vi "FilePackageReceive.vi"(8 "error in":errorcluster caption="错误输入（无错误）", 9 "PCFileLocation":string="C:\\Users\\Administrator\\Desktop\\Xmodem_2_FileReceive", 10 "PdFileLocation":string="/media/card/15CAG2018070200000025.key", 11 "ComIn":refnum<visa-resource-name>="COM16") -> (0 "error out":errorcluster caption="错误输出", 1 "Times":dbl, 2 "MD5":string, 3 "Result":bool, 4 "FileText":string, 5 "FileLen":u32)   [LabVIEW 2013]
uses:
  <vilib>/Instr/_visa.llb/VISA Flush IO Buffer Mask.ctl
  <vilib>/Instr/_visa.llb/VISA Set IO Buffer Mask.ctl
  RegisterPara.ctl
  <vilib>/Instr/_visa.llb/VISA Configure Serial Port (Instr).vi
  FileGolbalPara.vi
panel:
  out "数组":string[](array[string])
  out "MD5_2":string
  out "连接的字符串 2":string
  out "CRC？":bool
  out "文件内容":string
  out "读取缓冲区2":string
  out "连接的字符串":string
  out "FileName":string
  out "读取缓冲区":string
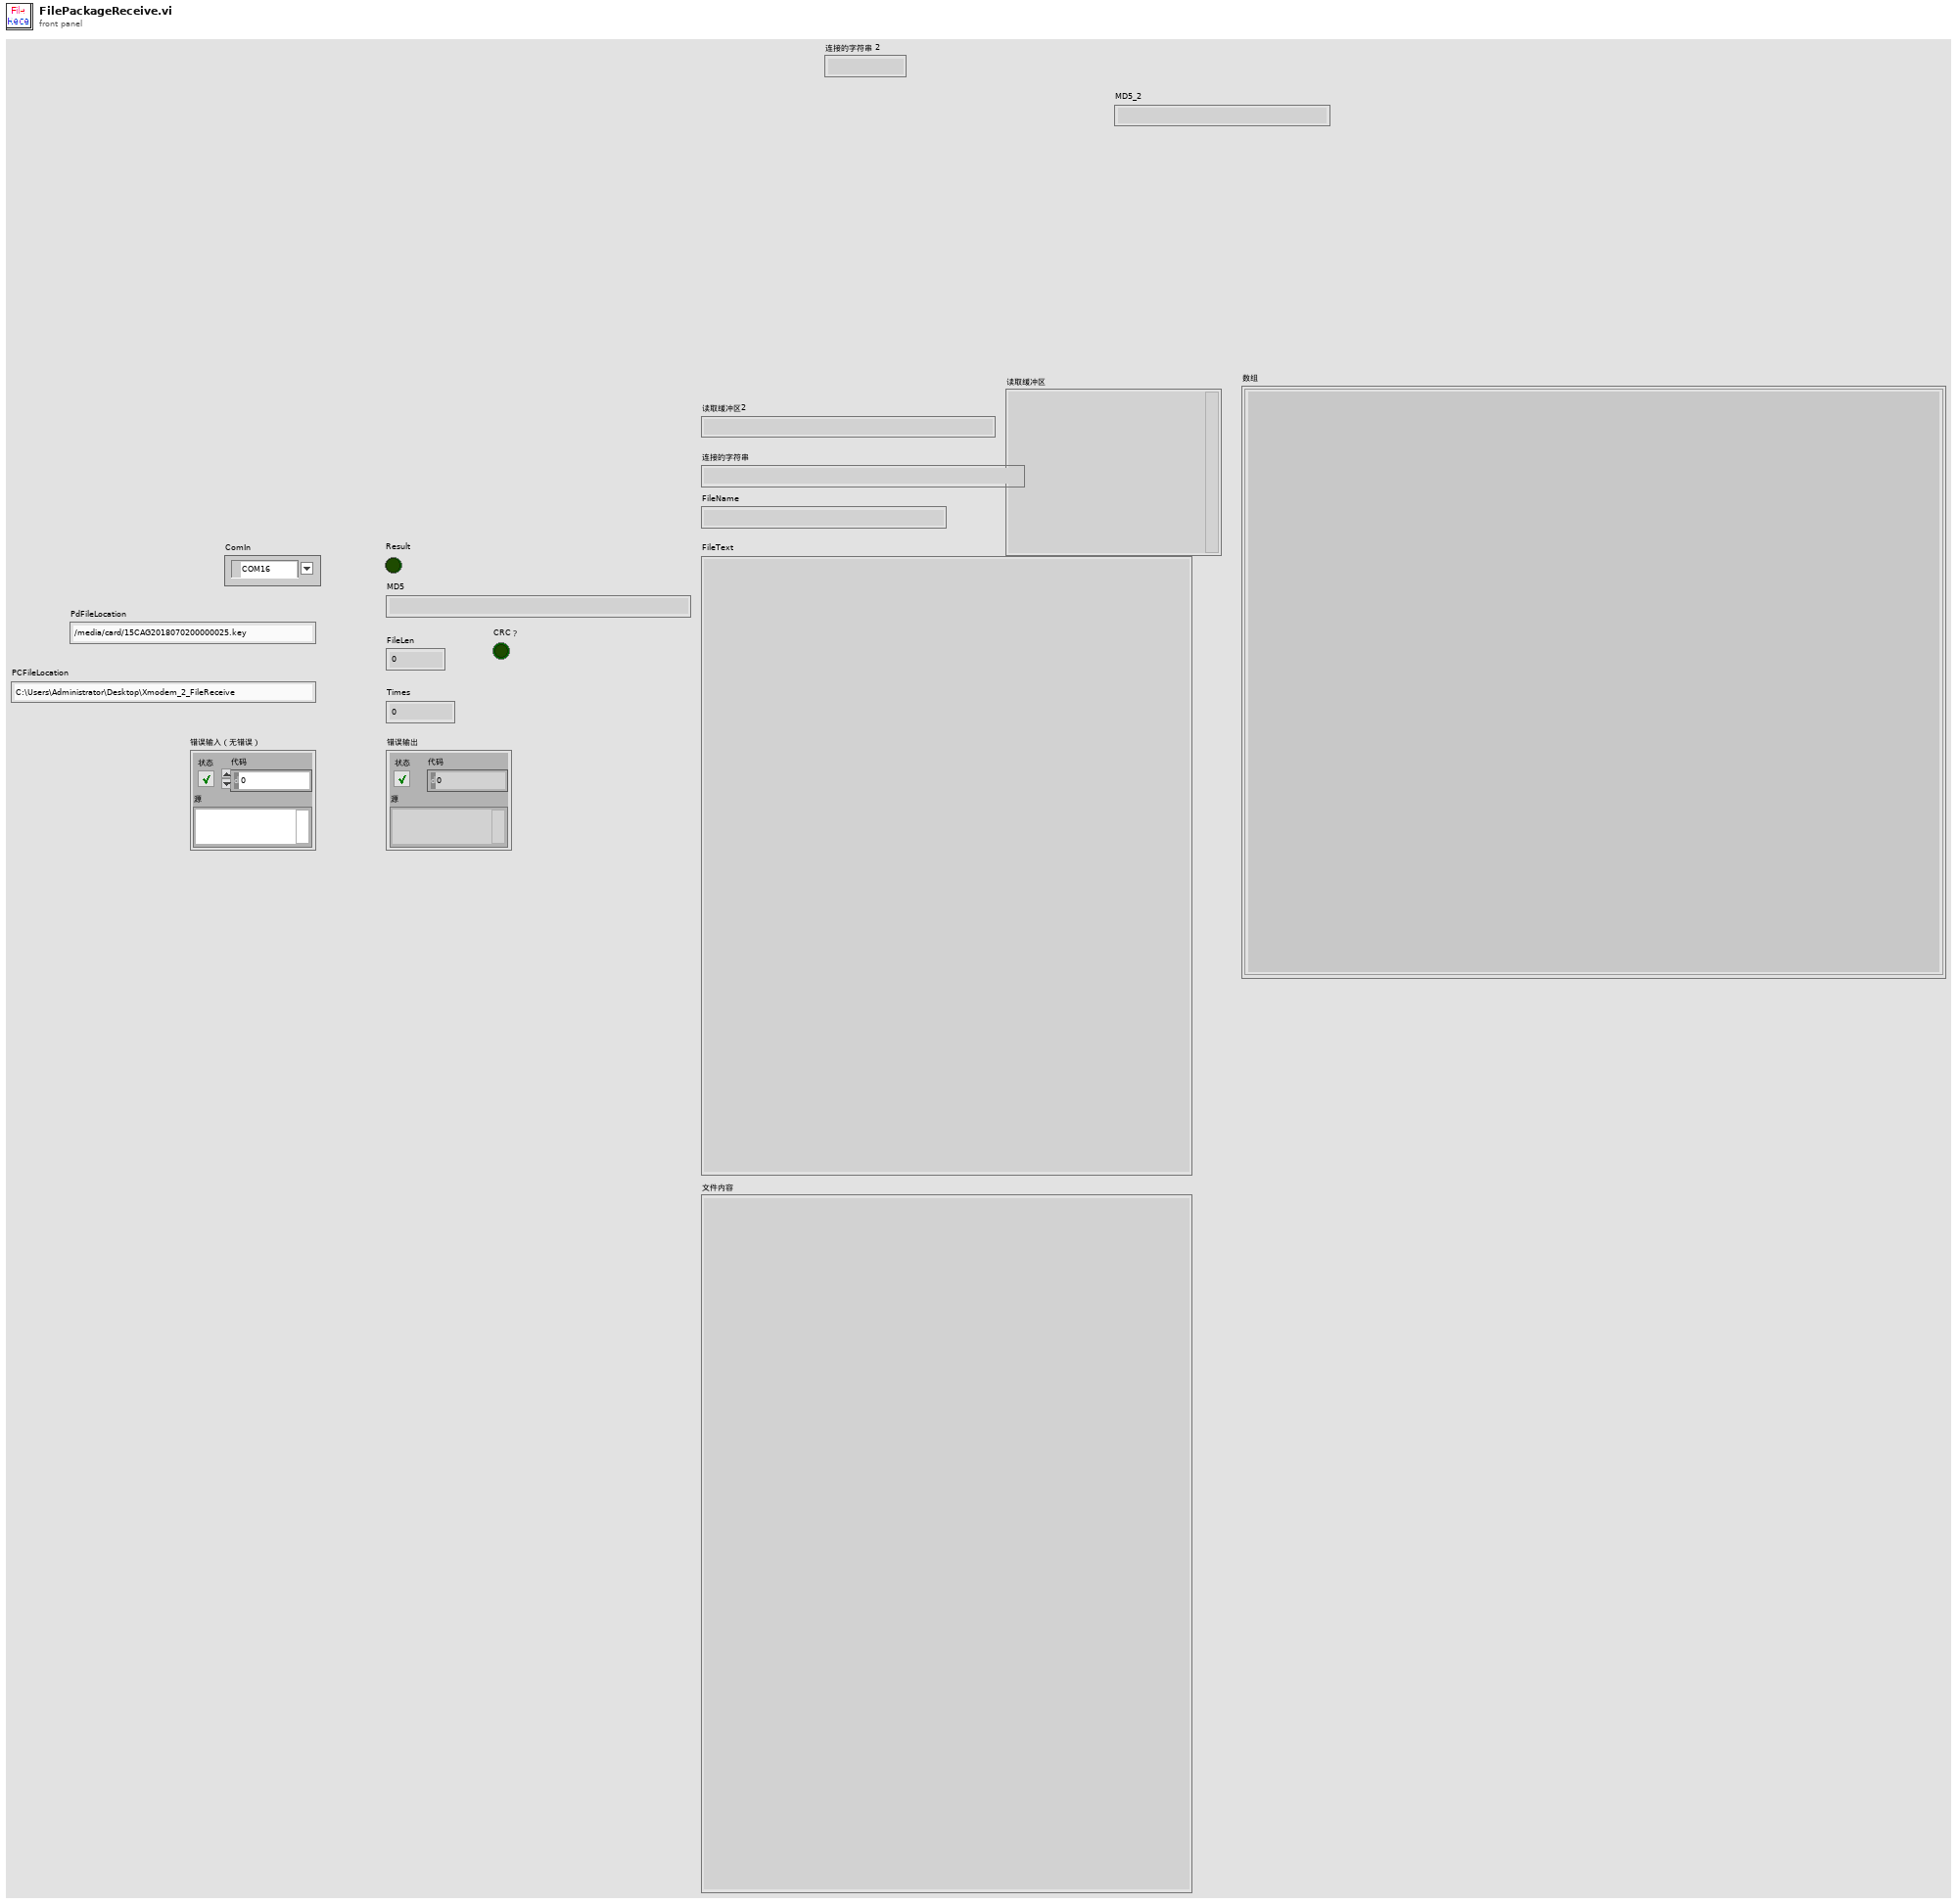
[diagram p1: front panel]
types:
  T1 = typedef "VISA Flush IO Buffer Mask.ctl" = u16
  T2 = cluster{"波特率":u32, "数据比特":u16, "奇偶":enum16{"None", "Odd", "Even", "Mark", "Space"}, "停止位":u16, "流控制":u16}
  T3 = typedef "RegisterPara.ctl" = cluster{"MD5":string, "文件总字节数":u32, "文件帧数":u32, "帧方式":enum16{"128K", "1024K-128K"}, "文件内容":string, "帧序号溢出标志":u32, "128包数":u32, "1024包数":u32}
  T4 = typedef "VISA Set IO Buffer Mask.ctl" = u16
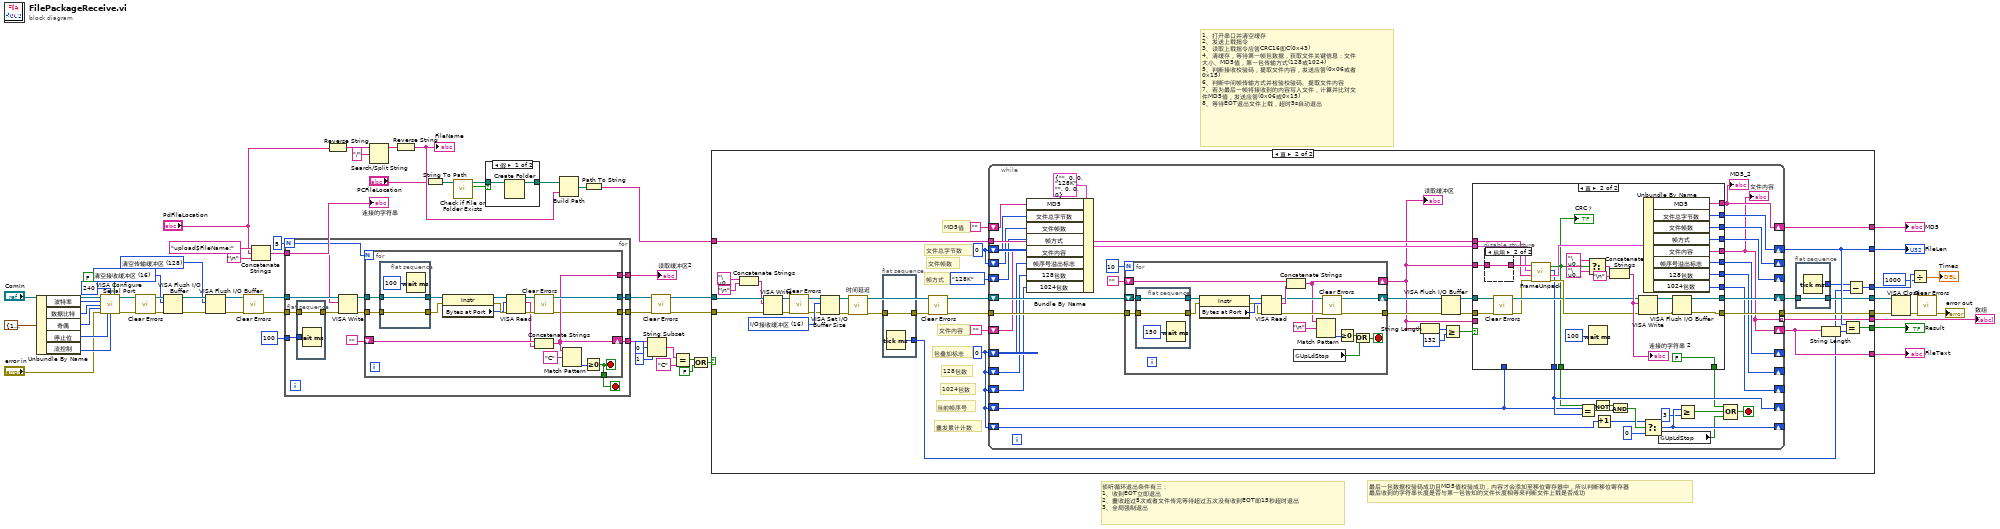
[diagram p0: block diagram]
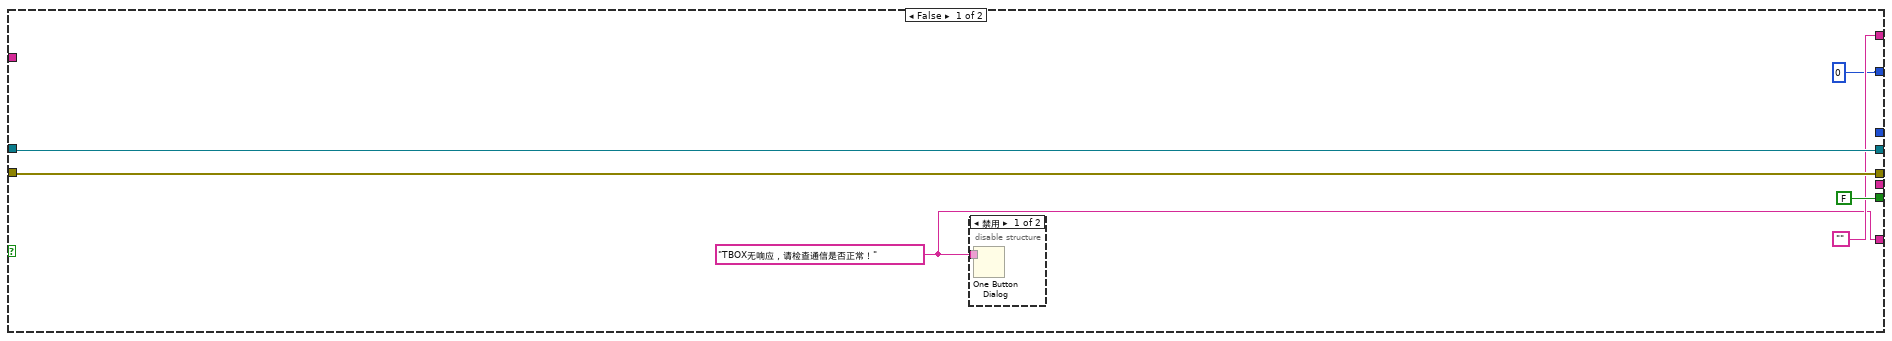
[diagram p3: hidden frame]
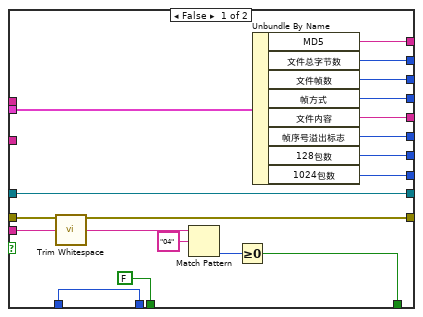
[diagram p5: hidden frame]
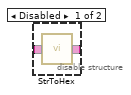
[diagram p6: hidden frame]
diagram:
  w48 = T1 128 items=["清空接收缓冲区"=16, "向设备写入传输缓冲区"=32, "清空接收缓冲区（无I/O）"=64, "清空传输缓冲区"=128] ("Mask")
  w52 = T1 16 items=["清空接收缓冲区"=16, "向设备写入传输缓冲区"=32, "清空接收缓冲区（无I/O）"=64, "清空传输缓冲区"=128] ("Mask")
  # "最后一包数据校验码成功且MD5值校验成功，内容才会添加至移位寄存器中，所以判断移位寄存器\n最后收到的字符串长度是否与第一包告知的文件长度相等来判断文件上载是否成功"
  # "侦听循环退出条件有三：\n1、收到EOT立即退出\n2、重收超过5次或者文件传完等待超过五次没有收到EOT即15秒超时退出\n3、全局强制退出"
  # "1、打开串口并清空缓存\n2、发送上载指令\n3、读取上载指令应答CRC16即C(0x43)\n4、清缓存，等待第一帧包数据，获取文件关键信息：文件\n大小、MD5值，第一包传输方式(128或1024)\n5、判断接收校验码，提取文件内容，发送应答(0x06或者\n0x15)\n6、判断中间帧传输方式并检验校验码、提取文件内容\n7、若为最后一帧将接收到的内容写入文件，计算并比对文\n件MD5值，发送应答(0x06或0x15)\n8、等待EOT退出文件上载，超时5s自动退出"
  n1 = Unbundle By Name(T2 {"波特率"=115200, "数据比特"=8, "奇偶"=enum."None", "停止位"=10, "流控制"=0} ("串口设置")) -> ("波特率"=w59:u32, "数据比特"=w58:u16, "奇偶"=w57:enum16{"None", "Odd", "Even", "Mark", "Space"}, "停止位"=w56:u16, "流控制"=w55:u16)
  n2 = call-poly "VISA Configure Serial Port"("VISA resource name"="ComIn", "termination char\n(0xA = '\\n' = LF)"=u8 240 ("termination char\n(0xA = '\\n' = LF)"), "Enable Termination\nChar (T)"=FALSE ("Enable Termination\nChar (T)"), "baud rate (9600)"=w59, "data bits (8)"=w58, "parity (0:none)"=w57, "error in (no error)"="error in", "stop bits (10: 1 bit)"=w56, "flow control (0:none)"=w55) -> ("VISA resource name out"=w53:refnum<visa-resource-name>, "error out"=w51:errorcluster)  [unwired: 5 in]
  n3 = call <vilib>:"Clear Errors.vi"("error in (no error)"=w51) -> ("error out"=w4:errorcluster)  [unwired: 6 in]
  n4 = VISA Flush I/O Buffer(VISA resource name=w53, mask (16)=w52, error in (no error)=w4) -> (VISA resource name out=w50:refnum<visa-resource-name>, error out=w49:errorcluster)
  n5 = VISA Flush I/O Buffer(VISA resource name=w50, mask (16)=w48, error in (no error)=w49) -> (VISA resource name out=w47:refnum<visa-resource-name>, error out=w46:errorcluster)
  n6 = call <vilib>:"Clear Errors.vi"("error in (no error)"=w46) -> ("error out"=w3:errorcluster)  [unwired: 6 in]
  n7 = Concatenate Strings("upload$FileName:", "PdFileLocation", "\n") -> (w41:string)
  "连接的字符串" <- w41
  n8 = for {
    N: 5 -> [w66]
    tunnel: w47 -> [w75]
    tunnel: w3 -> [w64]
    tunnel: [w72] -> w43
    tunnel: [w71] -> w42
    tunnel: w41 -> [w70]
    tunnel: [w69] -> w17
    tunnel: [w67] -> w12
    tunnel: 100 -> [w62]
    stop <- w65 stop-if-true
    n9 = flat-sequence {
      tunnel: w64 -> [w77]
      tunnel: [w77] -> w63
      tunnel: w62 -> [w76]
      frame #0 {
        n10 = Wait (ms)(milliseconds to wait=w76) -> ()  [unwired: 1 out]
      }
    }
    n11 = VISA Write(VISA resource name=w75, write buffer=w70, error in (no error)=w63) -> (VISA resource name out=w74:refnum<visa-resource-name>, error out=w73:errorcluster)  [unwired: 1 out]
    n12 = for {
      N: w66 -> [_]
      tunnel: w74 -> [w93]
      tunnel: w73 -> [w92]
      tunnel: [w86] -> w72
      tunnel: [w78] -> w71
      tunnel: [w80] -> w69
      shift-right: [w80] -> w67
      shift-left: "" -> [w84]
      tunnel: [w79] -> w65
      stop <- w79 stop-if-true
      n13 = flat-sequence {
        tunnel: w93 -> [w95]
        tunnel: w92 -> [w94]
        tunnel: [w95] -> w91
        tunnel: [w94] -> w90
        frame #0 {
          n14 = Wait (ms)(milliseconds to wait=u32 100 ("等待时间（毫秒）")) -> ()  [unwired: 1 out]
        }
      }
      n15 = property class="Instr"(reference=w91, error in=w90) -> (reference out=w87:refnum<visa-resource-name>, error out=w89:errorcluster, "Bytes at Port"=w88:u32)
      n16 = VISA Read(VISA resource name=w87, byte count=w88, error in (no error)=w89) -> (VISA resource name out=w86:refnum<visa-resource-name>, read buffer=w83:string, error out=w85:errorcluster)  [unwired: 1 out]
      n17 = Concatenate Strings(w84, w83) -> (w80:string)
      n18 = call <vilib>:"Clear Errors.vi"("error in (no error)"=w85) -> ("error out"=w78:errorcluster)  [unwired: 6 in]
      n19 = Match Pattern(string=w80, regular expression="C") -> (offset past match=w81:i32)  [unwired: 1 in, 3 out]
      n20 = Greater Or Equal To 0?(x=w81) -> (x >= 0?=w79:bool)
    }
  }
  "读取缓冲区2" <- w17
  n21 = Reverse String(1:"PdFileLocation") -> (0:w26:string)
  n22 = Search/Split String(string=w26, search string/char (-)="/") -> (substring before match=w25:string)  [unwired: 1 in, 2 out]
  n23 = Reverse String(1:w25) -> (0:w22:string)
  "FileName" <- w22
  n24 = String To Path(string="PCFileLocation") -> (path=w15:path)
  n25 = call <vilib>:"Check if File or Folder Exists.vi"("path"=w15) -> ("file or folder exists?"=w7:bool, "dup path"=w6:path)  [unwired: 8 in, 1 out]
  n26 = case shown="假" w7 {
    tunnel: w6 -> [w98 w99]
    tunnel: [w97 w99] -> w5
    frame False {
      n27 = Create Folder(path (use dialog)=w98) -> (created path=w97:path)  [unwired: 2 in, 2 out]
    }
    frame True {
    }
  }
  n28 = Build Path(base path=w5, name or relative path=w22) -> (appended path=w36:path)
  n29 = Path To String(path=w36) -> (string=w35:string)
  n30 = String Subset(string=w12, offset (0)=0 ("偏移量(0)"), length (rest)=1) -> (substring=w11:string)
  n31 = call <vilib>:"Clear Errors.vi"("error in (no error)"=w42) -> ("error out"=w2:errorcluster)  [unwired: 6 in]
  n32 = Equal?(x=w11, y="C") -> (x = y?=w40:bool)
  n33 = Or(x=w40, y=FALSE) -> (x .or. y?=w39:bool)
  n34 = case shown="真" w39 {
    tunnel: w43 -> [w105 w137]
    tunnel: w2 -> [w104 w136]
    tunnel: w35 -> [_ w132]
    tunnel: [w105 w112] -> w28
    tunnel: [w104 w131] -> w27
    tunnel: [FALSE w124] -> w34
    tunnel: [w100 w123] -> w33
    tunnel: ["" w122] -> w32
    tunnel: [u32 0 w121] -> w31
    tunnel: [_ w116] -> w21
    tunnel: [_ w109] -> w20
    frame False {
      w100 = "TBOX无响应，请检查通信是否正常！" ("消息")
      n35 = disable-structure shown="禁用" {
        disable-tunnel: w100 -> [w106 _]
        frame Disabled {
          n36 = One Button Dialog(message=w106) -> ()  [unwired: 1 in, 1 out]
        }
        frame Enabled {
        }
      }
    }
    frame True {
      w129 = u32 0
      w126 = u32 0
      w135 = T4 16 items=["I/O接收缓冲区"=16, "I/O传输缓冲区"=32, "I/O接收和传输缓冲区"=48] ("Mask")
      # "重发累计计数"
      # "当前帧序号"
      # "1024包数"
      # "128包数"
      # "文件内容"
      # "帧方式"
      # "文件帧数"
      # "包叠加标志"
      # "文件总字节数"
      # "MD5值"
      n37 = Concatenate Strings("\u0006", "\n") -> (w117:string)
      n38 = VISA Write(VISA resource name=w137, write buffer=w117) -> (VISA resource name out=w120:refnum<visa-resource-name>)  [unwired: 1 in, 2 out]
      n39 = call <vilib>:"Clear Errors.vi"("error in (no error)"=w136) -> ("error out"=w107:errorcluster)  [unwired: 6 in]
      n40 = VISA Set I/O Buffer Size(VISA resource name=w120, mask (16)=w135, error in (no error)=w107) -> (VISA resource name out=w134:refnum<visa-resource-name>, error out=w133:errorcluster)  [unwired: 1 in]
      n41 = call "时间延迟"("error in (no error)"=w133) -> ("error out"=w115:errorcluster)  [unwired: 10 in]
      n42 = flat-sequence {
        tunnel: w115 -> [w141]
        tunnel: [w141] -> w114
        tunnel: [w140] -> w110
        frame #0 {
          n43 = Tick Count (ms)() -> (millisecond timer value=w140:u32)
        }
      }
      n44 = call <vilib>:"Clear Errors.vi"("error in (no error)"=w114) -> ("error out"=w108:errorcluster)  [unwired: 6 in]
      n45 = while {
        tunnel: w108 -> [w187]
        tunnel: w132 -> [w183]
        tunnel: [w181] -> w131
        shift-right: [w180] -> w113
        shift-left: w134 -> [w188]
        shift-right: [w169] -> w122
        shift-left: "" -> [w178]
        shift-right: [w168] -> w121
        shift-left: w129 -> [w177]
        shift-right: [w165] -> _
        shift-left: w126 -> [w173]
        shift-right: [w167] -> _
        shift-left: w129 -> [w176]
        shift-right: [w166] -> _
        shift-left: enum16{"128K", "1024K-128K"}."128K" -> [w175]
        shift-right: [w143] -> w123
        shift-left: "" -> [w174]
        shift-right: [w164] -> _
        shift-left: w126 -> [w172]
        shift-right: [w163] -> _
        shift-left: w126 -> [w171]
        shift-right: [w161] -> _
        shift-left: w126 -> [w153]
        shift-right: [w148] -> _
        shift-left: w126 -> [w155]
        tunnel: [w143] -> w116 mode=indexing
        stop <- w144 stop-if-true
        n46 = Bundle By Name(cluster=T3 {"MD5"="", "文件总字节数"=0, "文件帧数"=0, "帧方式"=enum."128K", "文件内容"="", "帧序号溢出标志"=0, "128包数"=0, "1024包数"=0} ("RegisterOut"), "MD5"=w178, "文件总字节数"=w177, "文件帧数"=w176, "帧方式"=w175, "文件内容"=w174, "帧序号溢出标志"=w173, "128包数"=w172, "1024包数"=w171) -> (w170:T3)
        n47 = for {
          N: 10 -> [_]
          tunnel: w187 -> [w255]
          shift-right: [w241] -> w142
          shift-left: "" -> [w248]
          tunnel: [w239] -> w182
          shift-right: [w245] -> w184
          shift-left: w188 -> [w256]
          stop <- w243 stop-if-true
          n48 = flat-sequence {
            tunnel: w256 -> [w259]
            tunnel: [w259] -> w254
            tunnel: w255 -> [w257]
            tunnel: [w257] -> w252
            frame #0 {
              n49 = Wait (ms)(milliseconds to wait=u32 150 ("等待时间（毫秒）")) -> ()  [unwired: 1 out]
            }
          }
          n50 = property class="Instr"(reference=w254, error in=w252) -> (reference out=w253:refnum<visa-resource-name>, error out=w250:errorcluster, "Bytes at Port"=w251:u32)
          n51 = VISA Read(VISA resource name=w253, byte count=w251, error in (no error)=w250) -> (VISA resource name out=w245:refnum<visa-resource-name>, read buffer=w247:string, error out=w244:errorcluster)  [unwired: 1 out]
          n52 = Concatenate Strings(w248, w247) -> (w241:string)
          n53 = global read "FileGolbalPara.vi" "UpLdStop"() -> (w242:bool)
          n54 = Match Pattern(string=w241, regular expression="\n") -> (offset past match=w246:i32)  [unwired: 1 in, 3 out]
          n55 = call <vilib>:"Clear Errors.vi"("error in (no error)"=w244) -> ("error out"=w239:errorcluster)  [unwired: 6 in]
          n56 = Greater Or Equal To 0?(x=w246) -> (x >= 0?=w240:bool)
          n57 = Or(x=w240, y=w242) -> (x .or. y?=w243:bool)
        }
        "读取缓冲区" <- w142
        n58 = String Length(string=w142) -> (length=w152:i32)
        n59 = VISA Flush I/O Buffer(VISA resource name=w184) -> (VISA resource name out=w162:refnum<visa-resource-name>)  [unwired: 2 in, 1 out]
        n60 = Greater Or Equal?(x=w152, y=u32 132) -> (x >= y?=w151:bool)
        n61 = case shown="真" w151 {
          tunnel: w183 -> [_ w234]
          tunnel: w182 -> [w205 w233]
          tunnel: [w205 w210] -> w181
          tunnel: [w206 w208] -> w180
          tunnel: w142 -> [_ w231]
          tunnel: w170 -> [w204 w230]
          tunnel: [w203 w229] -> w169
          tunnel: [w202 w228] -> w168
          tunnel: [w201 w227] -> w167
          tunnel: [w200 w226] -> w166
          tunnel: [w199 w225] -> w143
          tunnel: [w198 w224] -> w165
          tunnel: [w197 w223] -> w164
          tunnel: [w196 w211] -> w163
          tunnel: w162 -> [w206 w215]
          tunnel: [w195 w214] -> w161
          tunnel: [FALSE w213] -> w158
          tunnel: w153 -> [w195 _]
          tunnel: w142 -> [w193 _]
          tunnel: [w189 FALSE] -> w149
          frame False {
            n62 = call <vilib>:"Trim Whitespace.vi"("string"=w193) -> ("trimmed string"=w192:string)  [unwired: 1 in]
            n63 = Match Pattern(string=w192, regular expression="04" ("正则表达式")) -> (offset past match=w190:i32)  [unwired: 1 in, 3 out]
            n64 = Greater Or Equal To 0?(x=w190) -> (x >= 0?=w189:bool)
            n65 = Unbundle By Name(w204) -> ("MD5"=w203:string, "文件总字节数"=w202:u32, "文件帧数"=w201:u32, "帧方式"=w200:enum16{"128K", "1024K-128K"}, "文件内容"=w199:string, "帧序号溢出标志"=w198:u32, "128包数"=w197:u32, "1024包数"=w196:u32)
          }
          frame True {
            n66 = disable-structure shown="启用" {
              disable-tunnel: [w237 w238] -> w235
              disable-tunnel: w231 -> [w236 w238]
              frame Disabled {
                n67 = call "StrToHex.vi"("StrIn"=w236) -> ("StrOut"=w237:string)
              }
              frame Enabled {
              }
            }
            n68 = call <vilib>:"Clear Errors.vi"("error in (no error)"=w233) -> ("error out"=w207:errorcluster)  [unwired: 6 in]
            n69 = call "FrameUnpack.vi"("error in"=w207, "FilePath"=w234, "RegisterIn"=w230, "FramePack"=w235) -> ("error out"=w216:errorcluster, "RegisterOut"=w222:T3, "当前接收包序号"=w214:u32, "CRC？"=w213:bool)  [unwired: 4 in]
            "CRC？" <- w213
            n70 = Select(t="\u0006", s=w213, f="\u0015") -> (s? t:f=w219:string)
            n71 = Wait (ms)(milliseconds to wait=u32 100 ("等待时间（毫秒）")) -> ()  [unwired: 1 out]
            n72 = Concatenate Strings(w219, "\n") -> (w217:string)
            "连接的字符串 2" <- w217
            n73 = VISA Write(VISA resource name=w215, write buffer=w217, error in (no error)=w216) -> (VISA resource name out=w232:refnum<visa-resource-name>, error out=w210:errorcluster)  [unwired: 1 out]
            n74 = Unbundle By Name(w222) -> ("MD5"=w229:string, "文件总字节数"=w228:u32, "文件帧数"=w227:u32, "帧方式"=w226:enum16{"128K", "1024K-128K"}, "文件内容"=w225:string, "帧序号溢出标志"=w224:u32, "128包数"=w223:u32, "1024包数"=w211:u32)
            n75 = VISA Flush I/O Buffer(VISA resource name=w232) -> (VISA resource name out=w208:refnum<visa-resource-name>)  [unwired: 2 in, 1 out]
          }
        }
        "文件内容" <- w143
        "MD5_2" <- w169
        n76 = Equal?(x=w153, y=w161) -> (x = y?=w160:bool)
        n77 = Not(x=w158) -> (.not. x?=w159:bool)
        n78 = Increment(x=w155) -> (x+1=w156:u32)
        n79 = And(x=w159, y=w160) -> (x .and. y?=w157:bool)
        n80 = Select(t=w156, s=w157, f=u32 0) -> (s? t:f=w148:u32)
        n81 = global read "FileGolbalPara.vi" "UpLdStop"() -> (w145:bool)
        n82 = Greater Or Equal?(x=w148, y=u32 3) -> (x >= y?=w146:bool)
        n83 = Compound Arithmetic op=OR(w149, w146, w145) -> (w144:bool)
      }
      n84 = flat-sequence {
        tunnel: w113 -> [w139]
        tunnel: [w139] -> w112
        tunnel: [w138] -> w111
        frame #0 {
          n85 = Tick Count (ms)() -> (millisecond timer value=w138:u32)
        }
      }
      n86 = String Length(string=w123) -> (length=w125:i32)
      n87 = Equal?(x=w121, y=w125) -> (x = y?=w124:bool)
      n88 = Subtract(x=w111, y=w110) -> (x-y=w109:u32)
    }
  }
  "Result" <- w34
  "FileText" <- w33
  "MD5" <- w32
  "FileLen" <- w31
  "数组" <- w21
  n89 = VISA Close(VISA resource name=w28, error in (no error)=w27) -> (error out=w29:errorcluster)
  n90 = Divide(x=w20, y=1000) -> (x/y=→"Times":dbl)
  n91 = call <vilib>:"Clear Errors.vi"("error in (no error)"=w29) -> ("error out"=→"error out":errorcluster)  [unwired: 6 in]
